vi "GetQX.vi"(2 "error in":errorcluster) -> (0 "error out":errorcluster, 1 "data":string)   [LabVIEW 2010]
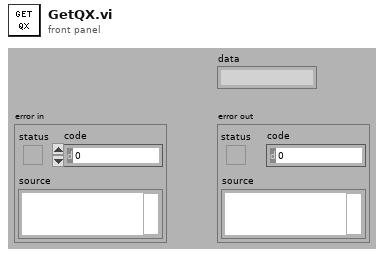
[diagram p1: front panel]
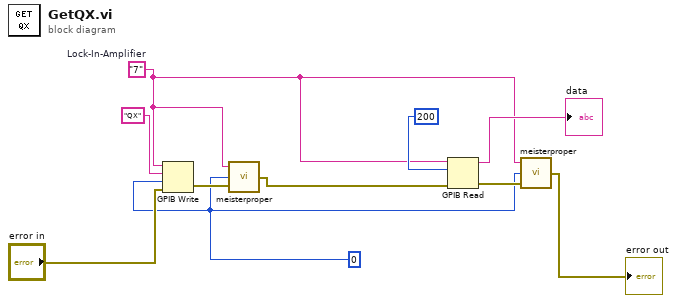
[diagram p0: block diagram]
diagram:
  w2 = i16 0 ("mode (0)")
  w1 = "7"  # Lock-In-Amplifier
  n1 = GPIB Write(0:w1, 1:"QX", 2:w2, 3:"error in") -> (6:w6:errorcluster)  [unwired: 1 in, 1 out]
  n2 = call "meisterproper.vi"("error in"=w6, "mode read"=w2, "adresse"=w1) -> ("error out"=w5:errorcluster)
  n3 = GPIB Read(0:w1, 1:200, 3:w5) -> (5:→"data":string, 7:w4:errorcluster)  [unwired: 2 in, 1 out]
  n4 = call "meisterproper.vi"("error in"=w4, "mode read"=w2, "adresse"=w1) -> ("error out"=→"error out":errorcluster)
